vi "Plot Loop.vi"(8 "error in":errorcluster, 9 "Cluster Of Graphs":T2, 10 "Reference For PLot":T3) -> (0 "error out":errorcluster)   [LabVIEW 2015]
uses:
  TypeDef/UE Reference For Plot.ctl
  TypeDef/Plot Cluster.ctl
  TypeDef/GraphReff.ctl
panel:
  in  "InitializationValue-Input-PieCahrt":T1={"InitializationDefect"=[0.0, 0.0, 0.0, 0.0, 0.0, 0.0, 0.0, 0.0, 0.0, 0.0, 0.0, 0.0, 0.0, 0.0, 0.0, 0.0, 0.0, 0.0, 0.0, 0.0, 0.0, 0.0, 0.0, 0.0, 0.0, 0.0, 0.0, 0.0, 0.0, 0.0, 0.0, 0.0, 0.0, 0.0, 0.0, 0.0, 0.0, 0.0, 0.0, 0.0], "InitializationProduction"=[0.0, 0.0, 0.0, 0.0, 0.0, 0.0, 0.0]}
  in  "InitializationValue-Input-Barplot":T1={"InitializationDefect"=[0.0, 0.0, 0.0, 0.0, 0.0, 0.0, 0.0, 0.0, 0.0, 0.0, 0.0, 0.0, 0.0, 0.0, 0.0, 0.0, 0.0, 0.0, 0.0, 0.0, 0.0, 0.0, 0.0, 0.0, 0.0, 0.0, 0.0, 0.0, 0.0, 0.0, 0.0, 0.0, 0.0, 0.0, 0.0, 0.0, 0.0, 0.0, 0.0, 0.0, 0.0], "InitializationProduction"=[0.0, 0.0, 0.0, 0.0, 0.0, 0.0]}
  # "Plot Loop Test Bench"
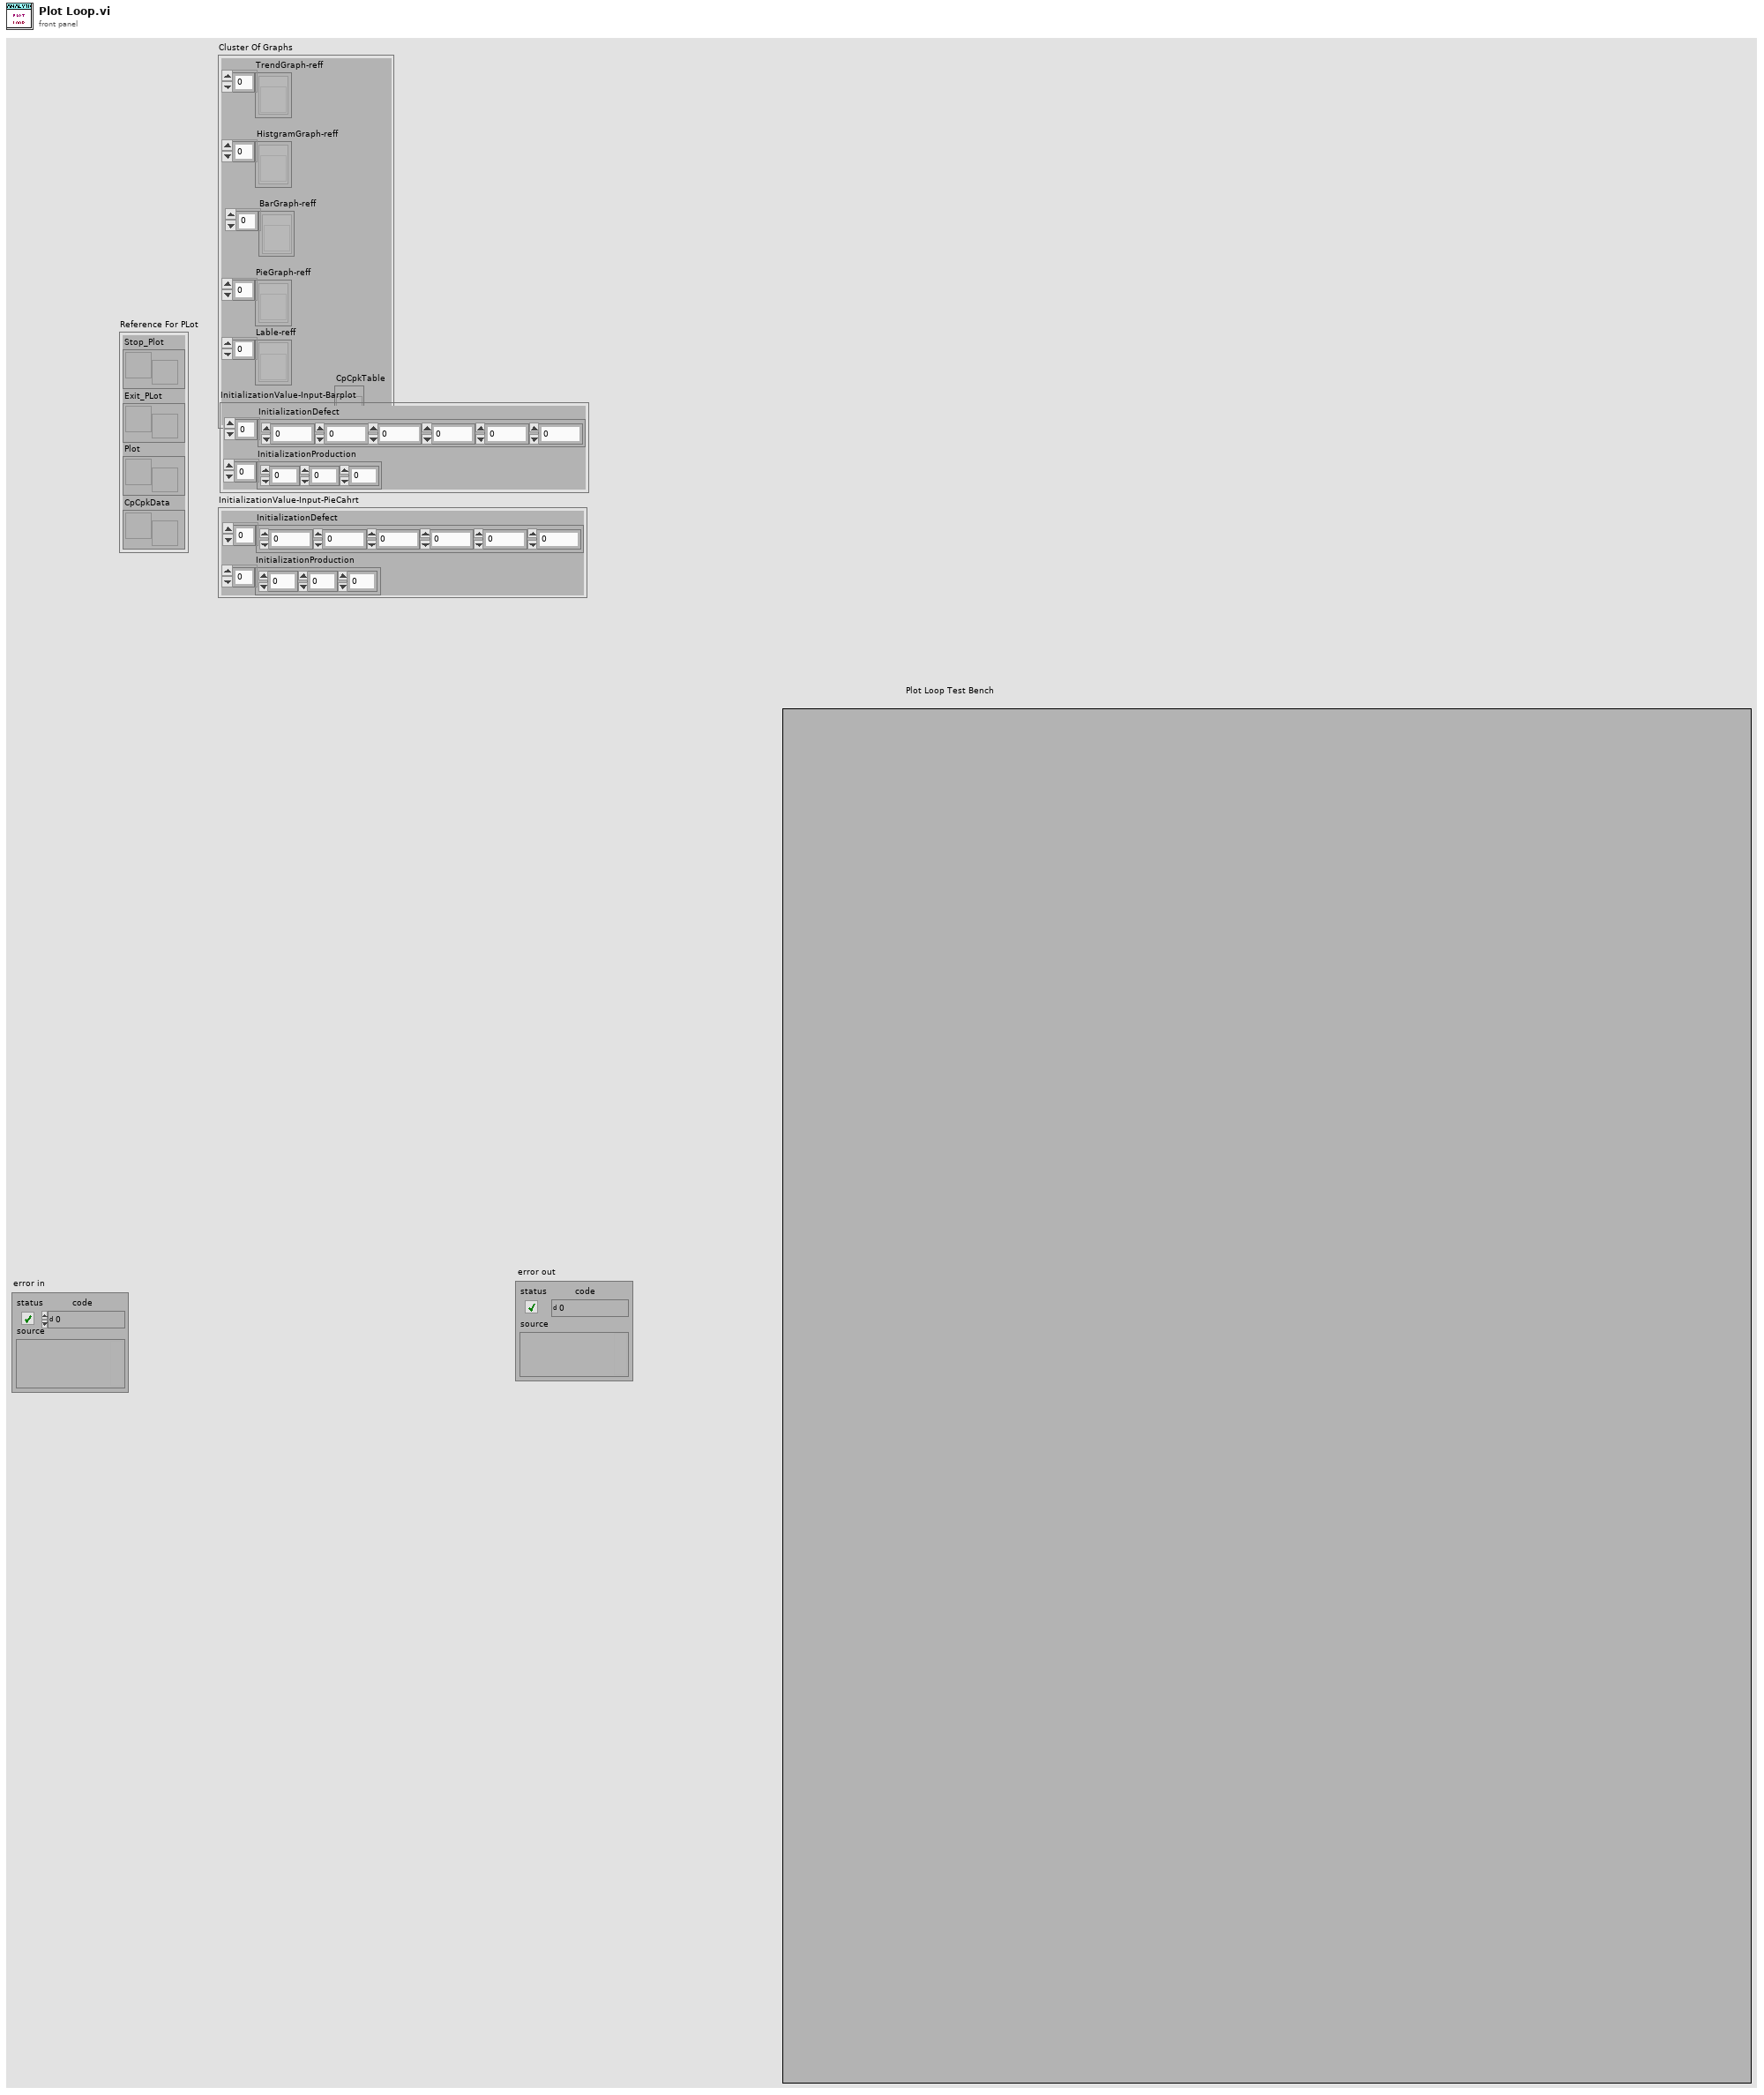
[diagram p1: front panel]
types:
  T1 = cluster{"InitializationDefect":dbl[], "InitializationProduction":dbl[]}
  T2 = typedef "GraphReff.ctl" = cluster{"HistgramGraph-reff":refnum<vi>[], "BarGraph-reff":refnum<vi>[], "PieGraph-reff":refnum<vi>[], "Lable-reff":refnum<vi>[], "TrendGraph-reff":refnum<vi>[], "CpCpkTable":refnum<vi>}
  T3 = typedef "UE Reference For Plot.ctl" = cluster{"Stop_Plot":refnum<user-event>, "Exit_PLot":refnum<user-event>, "Plot":refnum<user-event>, "CpCpkData":refnum<user-event>}
  T4 = enum32{"invalid app kind", "Development System", "Run Time System", "Student Edition", "Embedded LabVIEW", "Evaluation", "Custom"}
  T5 = enum32{"Invalid", "Standard", "Closed", "Hidden", "Minimized", "Maximized"}
  T6 = typedef "Plot Cluster.ctl" = cluster{"Reduced 2D":dbl[][], "Start Index":i32, "MeasurementData":cluster{"MeasurementID":i32, "MeasureEnable":bool, "MeasurementPass":bool, "LimitSets":cluster{"LimitSetId":i32, "Limits":dbl[]}[]}[], "No Of New Termnals":i32, "Top/Bottom":bool, "Values Inserted":i32, "PlotParameters":cluster{"Trend":cluster{"TrendID":i32, "PlotEnable":bool, "PlotTitle":string, "PlotCaptionFont":cluster{"FontName":string, "FontSize":i32, "IsBold":bool, "IsItalic":bool, "IsUnderline":bool, "IsStrikeout":bool, "FontColor":string}, "XLabel":string, "XLabelFont":cluster{"FontName":string, "FontSize":i32, "IsBold":bool, "IsItalic":bool, "IsUnderline":bool, "IsStrikeout":bool, "FontColor":string}, "SamplesToDisplay":i32, "Channels":cluster{"Label":string, "YLabelFont":cluster{"FontName":string, "FontSize":i32, "IsBold":bool, "IsItalic":bool, "IsUnderline":bool, "IsStrikeout":bool, "FontColor":string}, "MeasurementID":i32, "PlotColor":string, "PointShape":string, "ShowOnGraph":bool}[]}[], "Histogram":cluster{"HistogramID":i32, "PlotEnable":bool, "PlotTitle":string, "PlotLabelFont":cluster{"FontName":string, "FontSize":i32, "IsBold":bool, "IsItalic":bool, "IsUnderline":bool, "IsStrikeout":bool, "FontColor":string}, "XLabel":string, "XLabelFont":cluster{"FontName":string, "FontSize":i32, "IsBold":bool, "IsItalic":bool, "IsUnderline":bool, "IsStrikeout":bool, "FontColor":string}, "YLabel":string, "YLabelFont":cluster{"FontName":string, "FontSize":i32, "IsBold":bool, "IsItalic":bool, "IsUnderline":bool, "IsStrikeout":bool, "FontColor":string}, "MeasurementID":i32, "PlotColor":string, "SamplesToDisplay":i32}[], "BarPlot":cluster{"BarPlotID":i32, "BarValuesID":i32, "PlotEnable":bool, "PlotLabel":string, "PlotLabelFont":cluster{"FontName":string, "FontSize":i32, "IsBold":bool, "IsItalic":bool, "IsUnderline":bool, "IsStrikeout":bool, "FontColor":string}, "XLabel":string, "XLabelFont":cluster{"FontName":string, "FontSize":i32, "IsBold":bool, "IsItalic":bool, "IsUnderline":bool, "IsStrikeout":bool, "FontColor":string}, "YLabel":string, "YLabelFont":cluster{"FontName":string, "FontSize":i32, "IsBold":bool, "IsItalic":bool, "IsUnderline":bool, "IsStrikeout":bool, "FontColor":string}, "Sectors":string[]}[], "PieChart":cluster{"PieChartID":i32, "PieChartValueID":i32, "PlotEnable":bool, "PlotLabel":string, "PlotLabelFont":cluster{"FontName":string, "FontSize":i32, "IsBold":bool, "IsItalic":bool, "IsUnderline":bool, "IsStrikeout":bool, "FontColor":string}, "Sectors":string[]}[]}, "Re-Initialised":bool, "Statistical params":string[][], "MeasurementData_IndexValues":cluster{"Measurement-ID":i32[], "Measurement-Enable":bool[], "LSL":dbl[], "USL":dbl[]}}
  T7 = cluster{"MeasurementID":i32, "MeasureEnable":bool, "MeasurementPass":bool, "LimitSets":cluster{"LimitSetId":i32, "Limits":dbl[]}[]}[]
  T8 = cluster{"Trend":cluster{"TrendID":i32, "PlotEnable":bool, "PlotTitle":string, "PlotCaptionFont":cluster{"FontName":string, "FontSize":i32, "IsBold":bool, "IsItalic":bool, "IsUnderline":bool, "IsStrikeout":bool, "FontColor":string}, "XLabel":string, "XLabelFont":cluster{"FontName":string, "FontSize":i32, "IsBold":bool, "IsItalic":bool, "IsUnderline":bool, "IsStrikeout":bool, "FontColor":string}, "SamplesToDisplay":i32, "Channels":cluster{"Label":string, "YLabelFont":cluster{"FontName":string, "FontSize":i32, "IsBold":bool, "IsItalic":bool, "IsUnderline":bool, "IsStrikeout":bool, "FontColor":string}, "MeasurementID":i32, "PlotColor":string, "PointShape":string, "ShowOnGraph":bool}[]}[], "Histogram":cluster{"HistogramID":i32, "PlotEnable":bool, "PlotTitle":string, "PlotLabelFont":cluster{"FontName":string, "FontSize":i32, "IsBold":bool, "IsItalic":bool, "IsUnderline":bool, "IsStrikeout":bool, "FontColor":string}, "XLabel":string, "XLabelFont":cluster{"FontName":string, "FontSize":i32, "IsBold":bool, "IsItalic":bool, "IsUnderline":bool, "IsStrikeout":bool, "FontColor":string}, "YLabel":string, "YLabelFont":cluster{"FontName":string, "FontSize":i32, "IsBold":bool, "IsItalic":bool, "IsUnderline":bool, "IsStrikeout":bool, "FontColor":string}, "MeasurementID":i32, "PlotColor":string, "SamplesToDisplay":i32}[], "BarPlot":cluster{"BarPlotID":i32, "BarValuesID":i32, "PlotEnable":bool, "PlotLabel":string, "PlotLabelFont":cluster{"FontName":string, "FontSize":i32, "IsBold":bool, "IsItalic":bool, "IsUnderline":bool, "IsStrikeout":bool, "FontColor":string}, "XLabel":string, "XLabelFont":cluster{"FontName":string, "FontSize":i32, "IsBold":bool, "IsItalic":bool, "IsUnderline":bool, "IsStrikeout":bool, "FontColor":string}, "YLabel":string, "YLabelFont":cluster{"FontName":string, "FontSize":i32, "IsBold":bool, "IsItalic":bool, "IsUnderline":bool, "IsStrikeout":bool, "FontColor":string}, "Sectors":string[]}[], "PieChart":cluster{"PieChartID":i32, "PieChartValueID":i32, "PlotEnable":bool, "PlotLabel":string, "PlotLabelFont":cluster{"FontName":string, "FontSize":i32, "IsBold":bool, "IsItalic":bool, "IsUnderline":bool, "IsStrikeout":bool, "FontColor":string}, "Sectors":string[]}[]}
  T9 = cluster{"Measurement-ID":i32[], "Measurement-Enable":bool[], "LSL":dbl[], "USL":dbl[]}
  T10 = cluster{"Core":cluster{"Current VI Reference":refnum<vi>, "Close Panel on Exit?":bool}, "Plot-data":T6}
  T11 = cluster{"Current VI Reference":refnum<vi>, "Close Panel on Exit?":bool}
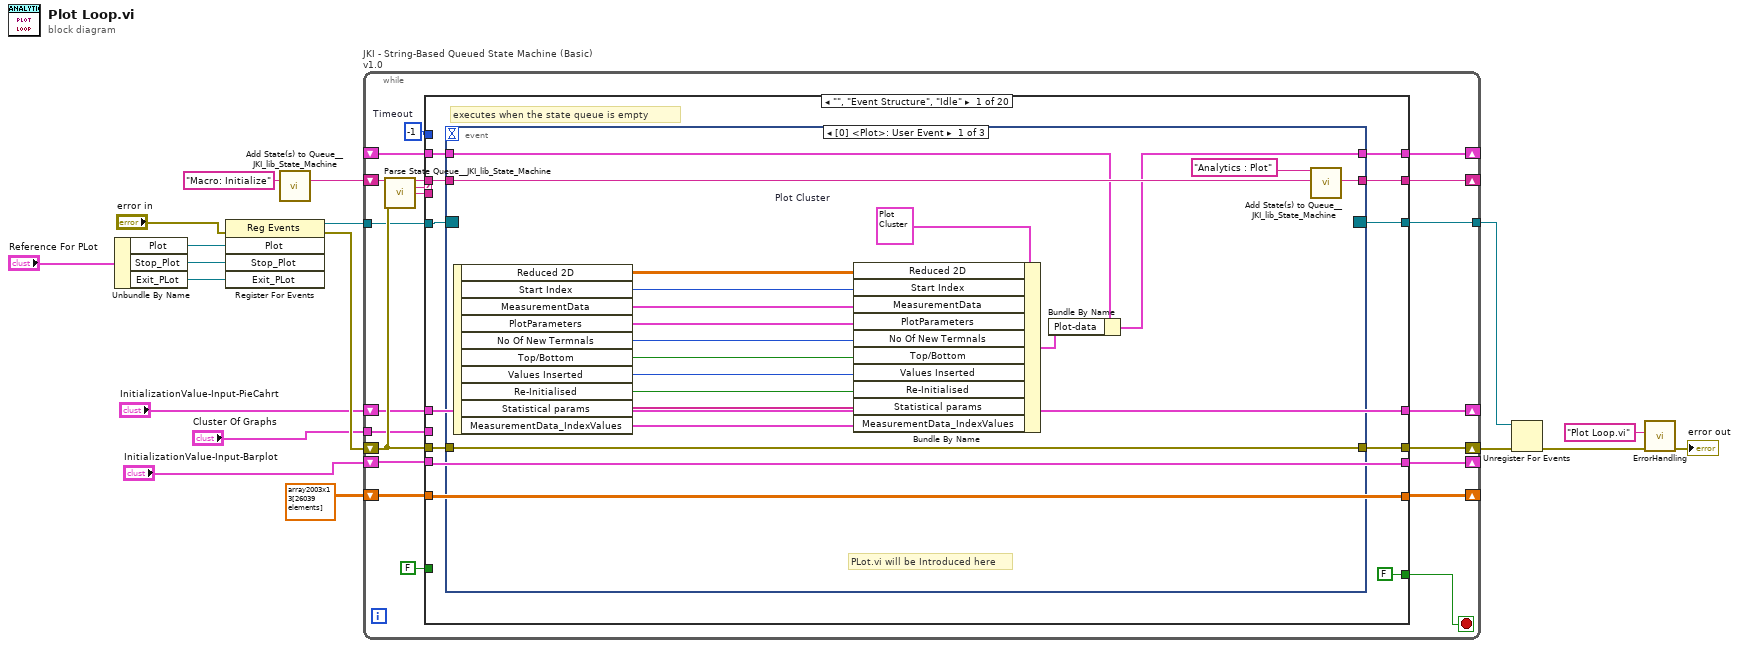
[diagram p0: block diagram]
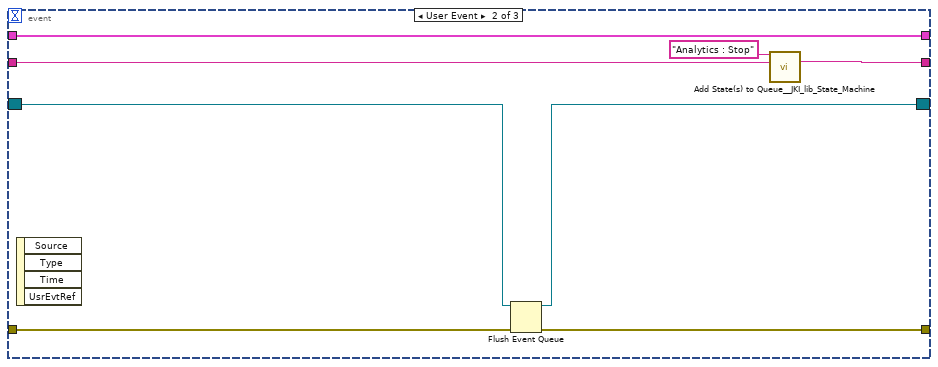
[diagram p2: hidden frame]
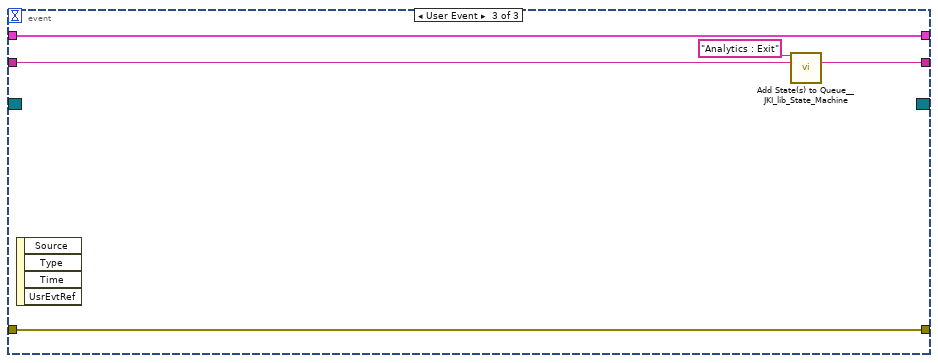
[diagram p3: hidden frame]
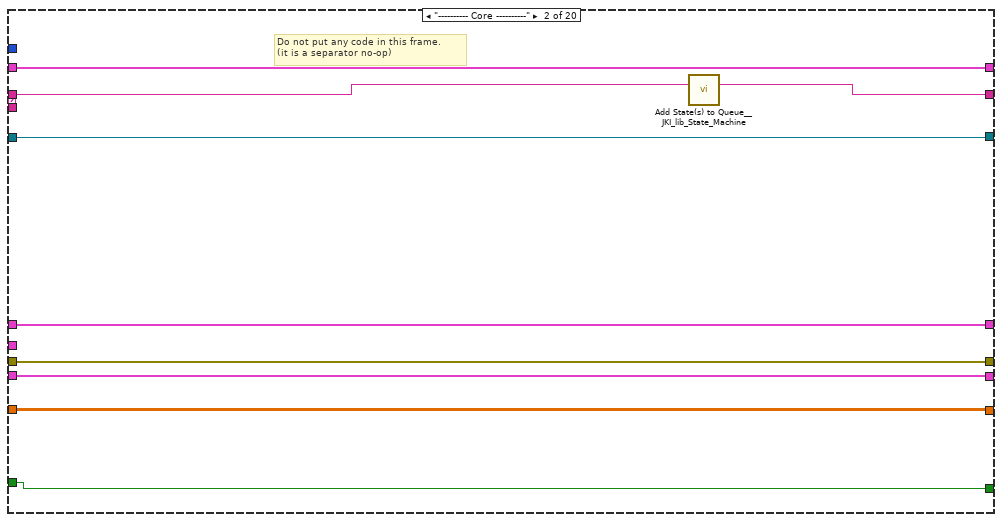
[diagram p4: hidden frame]
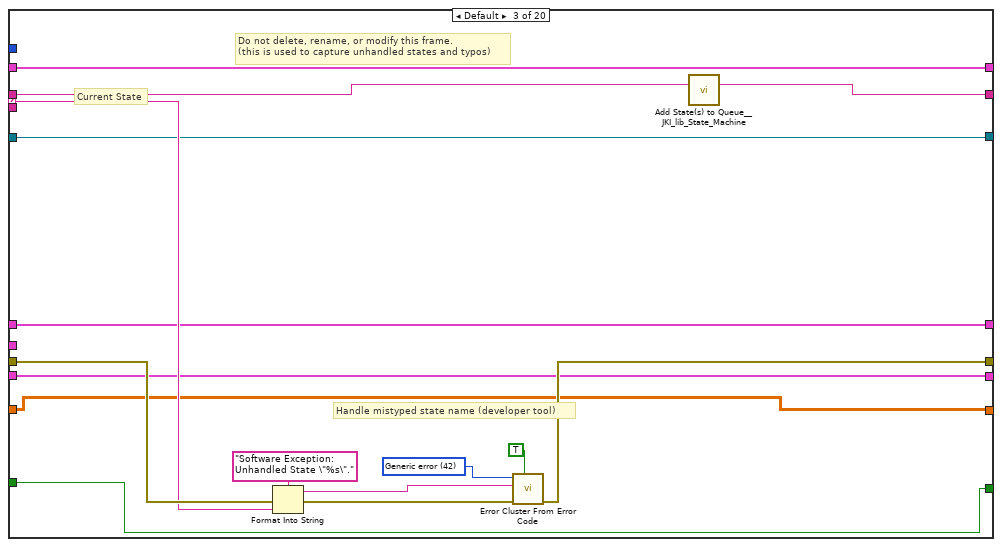
[diagram p5: hidden frame]
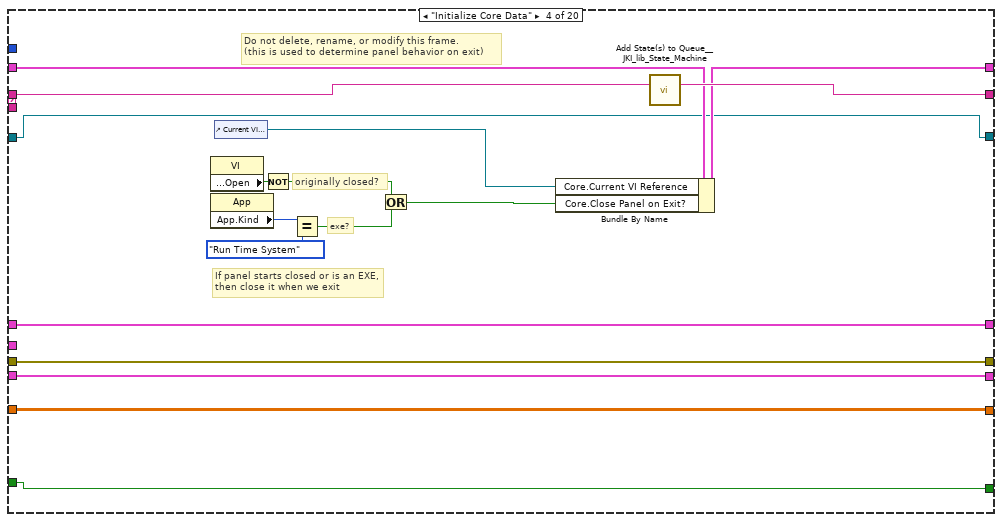
[diagram p6: hidden frame]
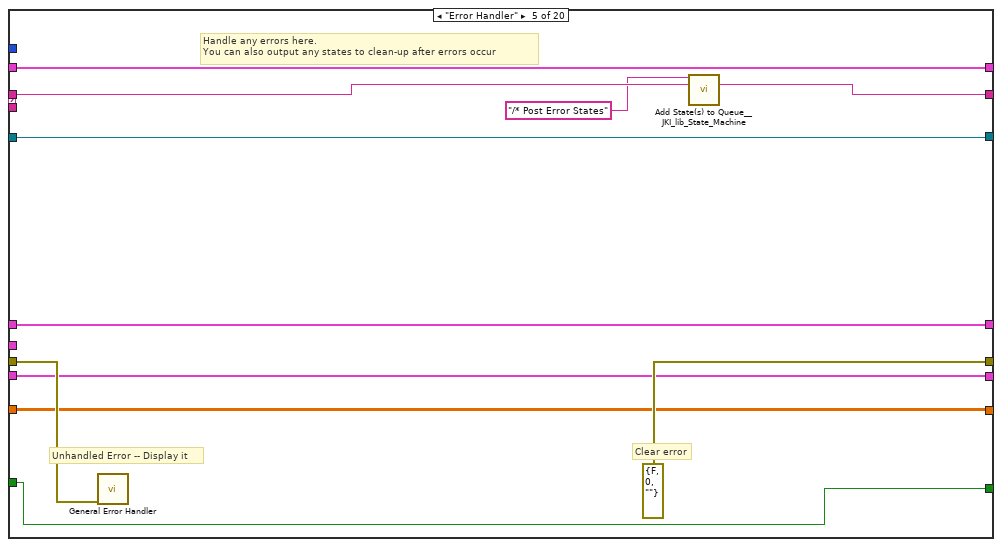
[diagram p7: hidden frame]
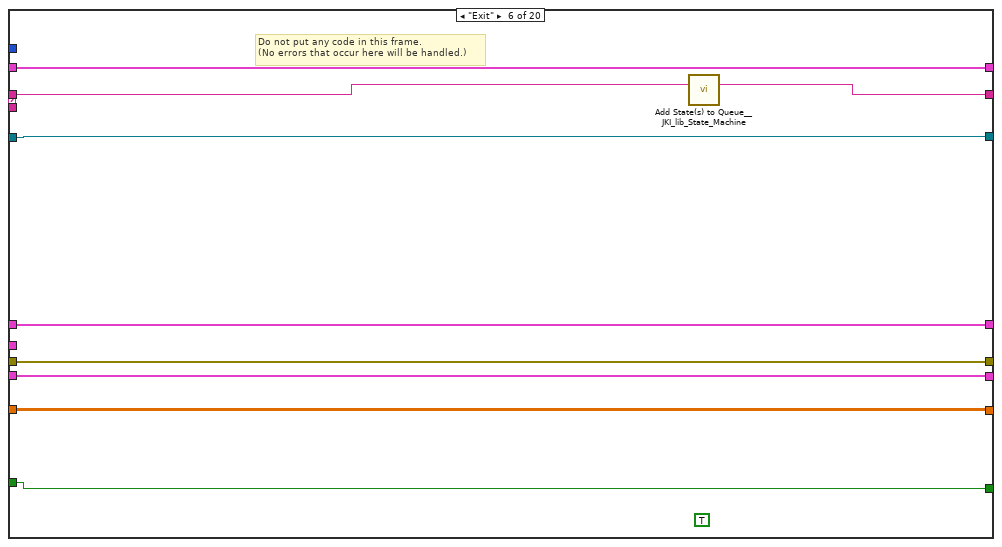
[diagram p8: hidden frame]
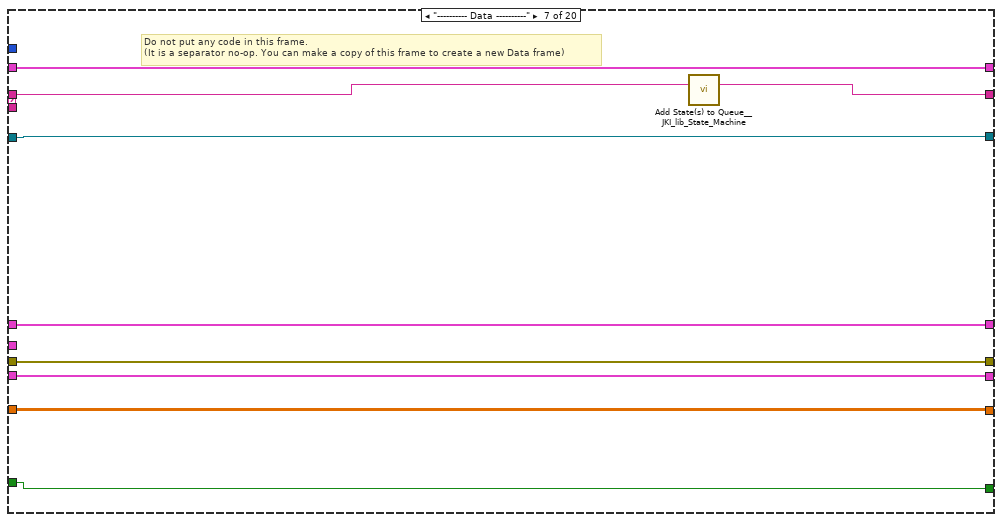
[diagram p9: hidden frame]
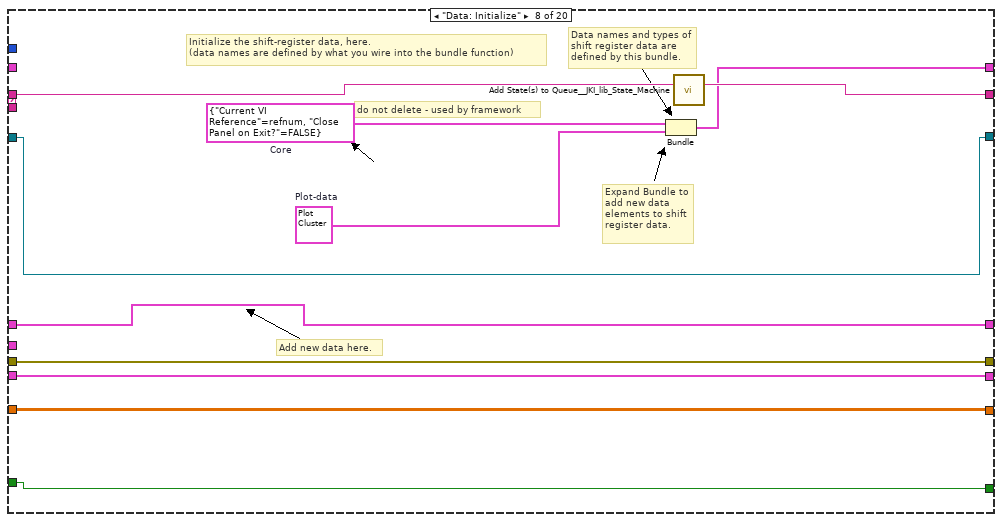
[diagram p10: hidden frame]
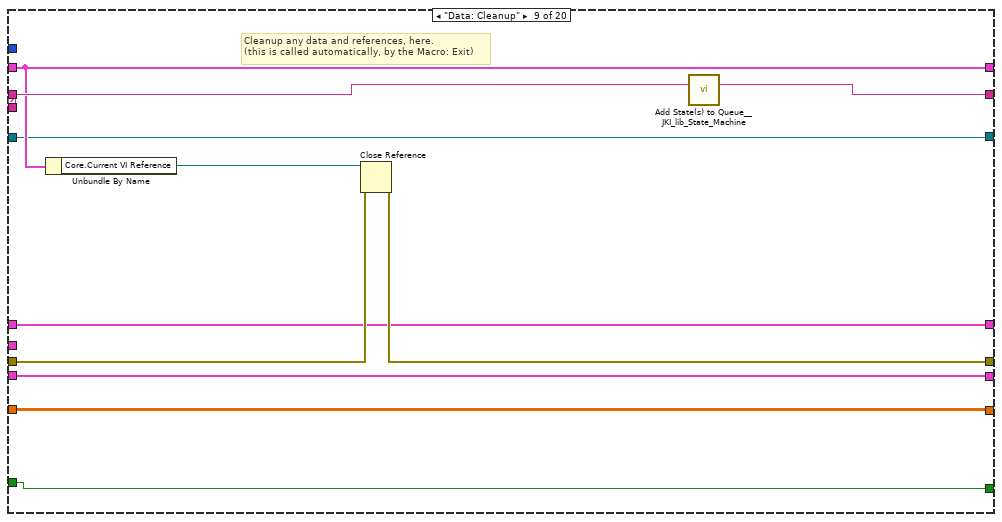
[diagram p11: hidden frame]
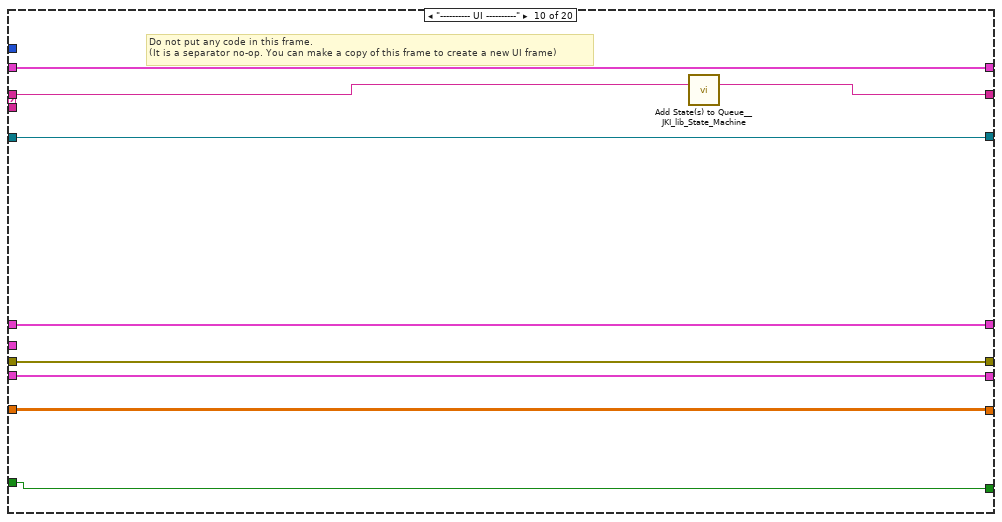
[diagram p12: hidden frame]
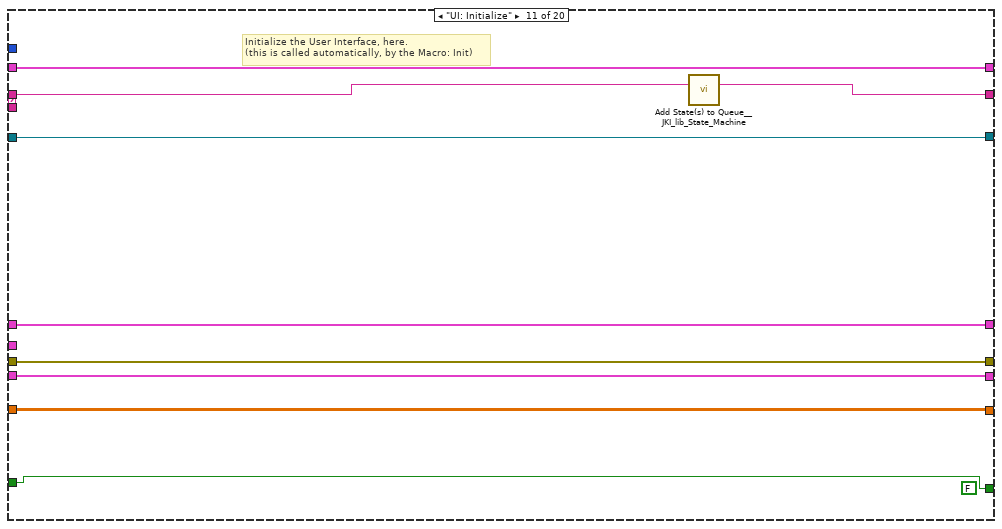
[diagram p13: hidden frame]
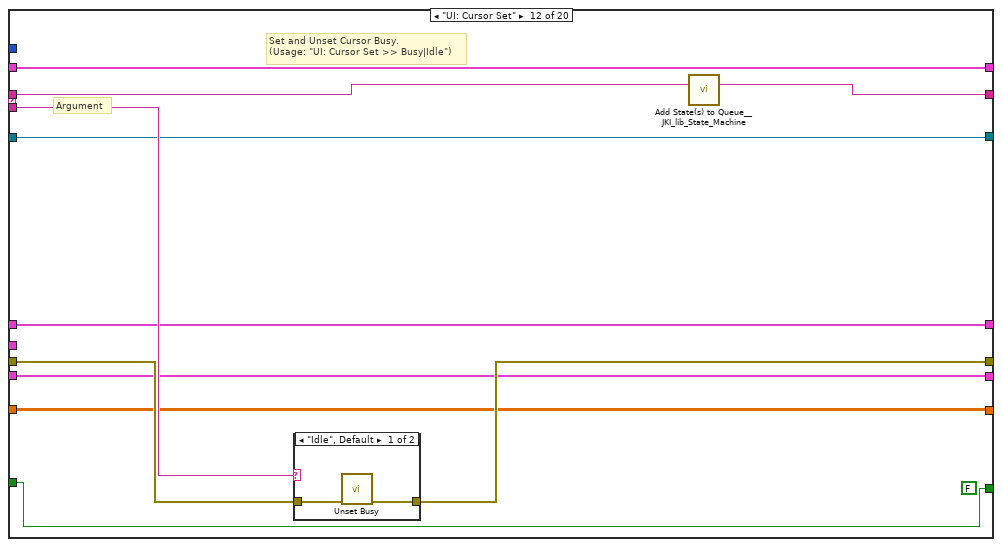
[diagram p14: hidden frame]
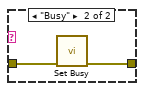
[diagram p15: hidden frame]
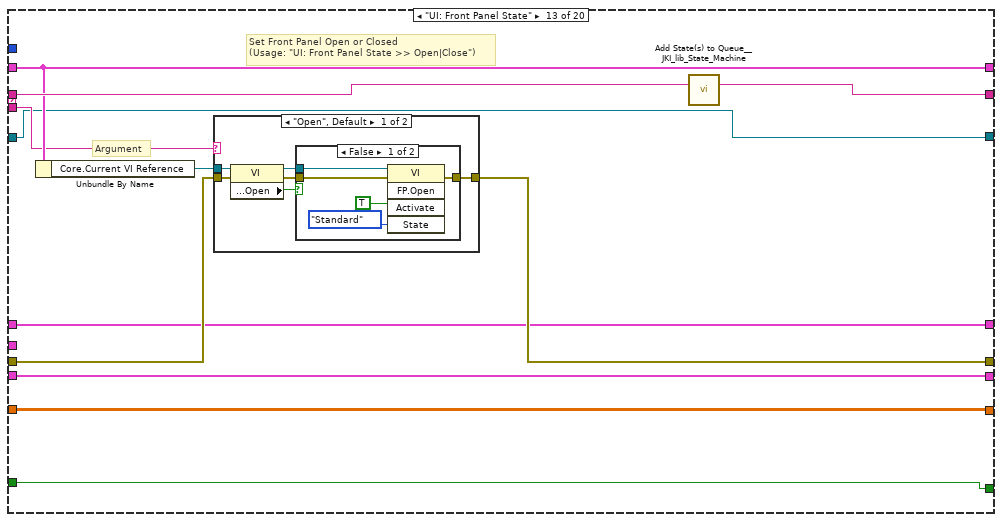
[diagram p16: hidden frame]
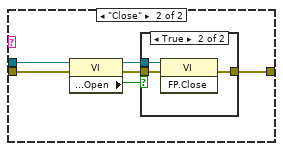
[diagram p18: hidden frame]
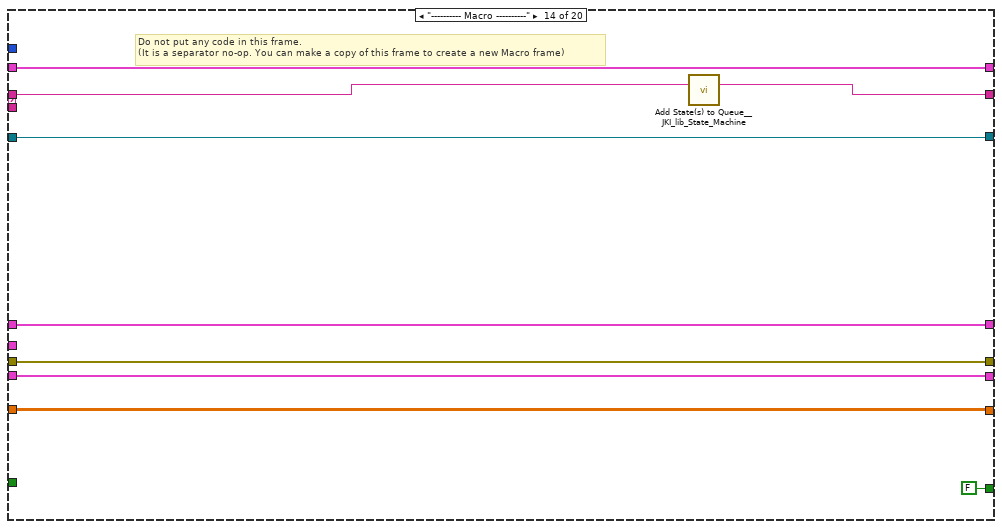
[diagram p20: hidden frame]
diagram:
  n1 = Unbundle By Name("Reference For PLot") -> ("Plot"=w11:refnum<user-event>, "Stop_Plot"=w15:refnum<user-event>, "Exit_PLot"=w14:refnum<user-event>)
  n2 = register-events(error in="error in", w11, w15, w14) -> (reference out=w8:refnum<event-registration>, error out=w7:errorcluster)  [unwired: 1 in]
  n3 = call <vilib>:"Add State(s) to Queue__JKI_lib_State_Machine.vi"("State(s) in (\"\")"="Macro: Initialize") -> ("States Out"=w10:string)  [unwired: 14 in]
  n4 = while "JKI - String-Based Queued State Machine (Basic) v1.0" {
    shift-right: [w33] -> _
    shift-left: _ -> [w32]
    shift-right: [w35] -> w2
    shift-left: w7 -> [w30]
    shift-right: [w34] -> _
    shift-left: w10 -> [w36]
    tunnel: w8 -> [w29]
    tunnel: "Cluster Of Graphs" -> [w26]
    tunnel: [w24] -> w1
    shift-right: [w22] -> _
    shift-left: "InitializationValue-Input-PieCahrt" -> [w25]
    shift-right: [w21] -> _
    shift-left: "InitializationValue-Input-Barplot" -> [w27]
    shift-right: [w23] -> _
    shift-left: dbl[][] array2003x13[26039 elements] ("Initialization input") -> [w28]
    stop <- w20 stop-if-true
    w31 = -1  # Timeout
    n5 = call <vilib>:"Parse State Queue__JKI_lib_State_Machine.vi"("State Queue"=w36, "Error In (no error)"=w30) -> ("Remaining States"=w38:string, "Current State"=w39:string, "Arguments"=w37:string)  [unwired: 11 in]
    n6 = case shown="\"\", \"Event Structure\", \"Idle\"" w39 {
      selector: w39 -> [_ _ w97 _ _ _ _ _ _ _ _ _ _ _ _ _ _ _ _ _]
      tunnel: w38 -> [w48 w91 w101 w124 w135 w144 w153 w164 w175 w184 w193 w204 w220 w251 w261 w276 w285 w300 w308 w310]
      tunnel: w37 -> [_ _ _ _ _ _ _ _ _ _ _ w199 w214 _ _ _ _ _ _ _]
      tunnel: w32 -> [w45 w88 w99 w115 w132 w142 w150 _ w170 w181 w191 w202 w216 w248 w258 w273 w282 w297 w305 w318]
      tunnel: [w50 w89 w103 w121 errorcluster {"status"=FALSE, "code"=0, "source"=""} ("error out") w141 w151 w161 w171 w182 w190 w200 w217 w249 w259 w274 w283 w295 w306 w315] -> w35
      tunnel: w30 -> [w51 w89 w102 w121 w131 w141 w151 w161 w172 w182 w190 w201 w218 w249 w259 w274 w283 w296 w306 w316]
      tunnel: [w47 w90 w100 w123 w134 w143 w152 w163 w174 w183 w192 w203 w219 w250 w260 w275 w284 w299 w307 w309] -> w34
      tunnel: [w46 w88 w99 w122 w132 w142 w150 w162 w170 w181 w191 w202 w216 w248 w258 w273 w282 w297 w305 w318] -> w33
      tunnel: w31 -> [_ _ _ _ _ _ _ _ _ _ _ _ _ _ _ _ _ _ _ _]
      tunnel: w29 -> [w49 w87 w96 w112 w129 w140 w149 w159 w169 w180 w189 w198 w213 w247 w256 w266 w281 w298 w304 w317]
      tunnel: w28 -> [w41 w84 w93 w109 w126 w137 w146 w155 w166 w177 w186 w195 w210 w244 w253 w263 w278 w291 _ _]
      tunnel: w27 -> [w40 w85 w94 w110 w127 w138 w147 w156 w167 w178 w187 w196 w211 w245 w254 w264 w279 w290 _ _]
      tunnel: w26 -> [_ _ _ _ _ _ _ _ _ _ _ _ _ _ _ _ _ w292 _ w314]
      tunnel: w25 -> [w42 w86 w95 w111 w128 w139 w148 w157 w168 w179 w188 w197 w212 w246 w255 w265 w280 w293 _ _]
      tunnel: [w44 w87 w96 w112 w129 w140 w149 w159 w169 w180 w189 w198 w213 w247 w256 w266 w281 w298 w304 w317] -> w24
      tunnel: [w41 w84 w93 w109 w126 w137 w146 w155 w166 w177 w186 w195 w210 w244 w253 w263 w278 w289 dbl[][] array2001x13[26013 elements] ("Initialization input") dbl[][] array2001x13[26013 elements] ("Initialization input")] -> w23
      tunnel: [w42 w86 w95 w111 w128 w139 w148 w157 w168 w179 w188 w197 w212 w246 w255 w265 w280 w288 w302 w313] -> w22
      tunnel: [w40 w85 w94 w110 w127 w138 w147 w156 w167 w178 w187 w196 w211 w245 w254 w264 w279 w287 w302 w313] -> w21
      tunnel: [FALSE w83 w92 w108 w125 w136 w145 w154 w165 w176 w185 w194 w209 FALSE FALSE TRUE FALSE FALSE FALSE TRUE] -> w20
      tunnel: FALSE -> [_ w83 w92 w108 w125 w136 w145 w154 w165 w176 w185 w194 w209 _ _ _ _ _ _ _]
      frame "", "Event Structure", "Idle" {
        # "executes when the state queue is empty"
        n7 = event shown="[0] <Plot>: User Event" {
          selector: w49 -> [_ w75 _]
          dyn-events: [_ w74 _] -> w44
          timeout: _ -> [_ _ _]
          tunnel: w51 -> [w57 w77 w78]
          tunnel: [w57 w76 w78] -> w50
          tunnel: w48 -> [w60 w71 w80]
          tunnel: [w59 w72 w81] -> w47
          tunnel: [w54 w73 w82] -> w46
          tunnel: w45 -> [w56 w73 w82]
          event User Event {
            w65 = T6 {"Reduced 2D"=[], "Start Index"=0, "MeasurementData"=[], "No Of New Termnals"=0, "Top/Bottom"=FALSE, "Values Inserted"=0, "PlotParameters"={"Trend"=[], "Histogram"=[], "BarPlot"=[], "PieChart"=[]}, "Re-Initialised"=FALSE, "Statistical params"=[], "MeasurementData_IndexValues"={"Measurement-ID"=[], "Measurement-Enable"=[], "LSL"=[], "USL"=[]}}  # Plot Cluster
            # "PLot.vi will be Introduced here"
            n8 = event-data() -> ("Reduced 2D"=w67:dbl[][], "Start Index"=w68:i32, "MeasurementData"=w66:T7, "PlotParameters"=w69:T8, "No Of New Termnals"=w64:i32, "Top/Bottom"=w63:bool, "Values Inserted"=w62:i32, "Re-Initialised"=w61:bool, "Statistical params"=w53:string[][], "MeasurementData_IndexValues"=w52:T9)  [unwired: 1 in]
            n9 = Bundle By Name(cluster=w65, "Reduced 2D"=w67, "Start Index"=w68, "MeasurementData"=w66, "PlotParameters"=w69, "No Of New Termnals"=w64, "Top/Bottom"=w63, "Values Inserted"=w62, "Re-Initialised"=w61, "Statistical params"=w53, "MeasurementData_IndexValues"=w52) -> (w55:T6)
            n10 = Bundle By Name(cluster=w56, "Plot-data"=w55) -> (w54:T10)
            n11 = call <vilib>:"Add State(s) to Queue__JKI_lib_State_Machine.vi"("State(s) in Front (\"\")"="Analytics : Plot" ("State(s) in Front (\"\")"), "State(s) in (\"\")"=w60) -> ("States Out"=w59:string)  [unwired: 13 in]
          }
          event User Event {
            n12 = event-data() -> ()  [unwired: 1 in, 4 out]
            n13 = Flush Event Queue(0:w75, 3:w77) -> (8:w74:refnum<event-registration>, 11:w76:errorcluster)  [unwired: 4 in, 1 out]
            n14 = call <vilib>:"Add State(s) to Queue__JKI_lib_State_Machine.vi"("State(s) in Front (\"\")"="Analytics : Stop" ("State(s) in Front (\"\")"), "State(s) in (\"\")"=w71) -> ("States Out"=w72:string)  [unwired: 13 in]
          }
          event User Event {
            n15 = event-data() -> ()  [unwired: 1 in, 4 out]
            n16 = call <vilib>:"Add State(s) to Queue__JKI_lib_State_Machine.vi"("State(s) in Front (\"\")"="Analytics : Exit" ("State(s) in Front (\"\")"), "State(s) in (\"\")"=w80) -> ("States Out"=w81:string)  [unwired: 13 in]
          }
        }
      }
      frame "---------- Core ----------" {
        # "Do not put any code in this frame.\n(it is a separator no-op)"
        n17 = call <vilib>:"Add State(s) to Queue__JKI_lib_State_Machine.vi"("State(s) in (\"\")"=w91) -> ("States Out"=w90:string)  [unwired: 14 in]
      }
      frame Default {
        w106 = 42 items=["No error", "Argument error", "Memory is full", "Out of zone", "End of file", "File already open", "Generic file I/O error", "File not found", "File permission error", "Disk is full", "Duplicate path", "Too many files open", "System feature not enabled", "Resource file not found", "Cannot add resource", "Resource not found", "Image not found", "Image memory error", "Pen does not exist", "Config type invalid", "Config token not found", "Config parse error", "Config memory error", "Bad external code format", "Bad external code offset", "External code not present", "Null window", "Destroy window error", "Null menu", "Print aborted", "Bad print record", "Print driver error", "Windows error during printing", "Memory error during printing", "Print dialog error", "Generic print error", "Invalid device refnum", "Device not found", "Device parameter error", "Device unit error", "Cannot open device", "Device call aborted", "Generic error", "Cancelled by user", "Object ID too low", "Object ID too high", "Object not in heap", "Unknown heap", "Unknown object (invalid DefProc)", "Unknown object (DefProc not in table)", "Message out of range", "Invalid (null) method", "Unknown message", "Manager call not supported", "Bad address", "Network operation in progress", "Network operation timed out", "Connection is busy", "Network attribute not supported", "Network error", "Address in use", "System out of memory", "Connection aborted", "Connection refused", "Not connected", "Already connected", "Connection closed", "Initialization error (interapplication manager)", "Bad occurrence", "Wait on unbound occurrence handler", "Occurrence queue overflow", "Datalog type conflict", "Unused", "Unrecognized type (interapplication manager)", "Memory corrupt", "Failed to make temporary DLL", "Old CIN version", "Drag socket not found", "Failed to load drop-object", "Failed to register OLE object", "Failed to release OLE object", "Format specifier type mismatch", "Unknown format specifier", "Too few format specifiers", "Too many format specifiers", "Scan failed", "Newer CIN version", "Error converting to variant", "Runtime menu error", "Password tampered", "Variant attribute not found", "Incompatible variant data type", "Event data is not available", "Event Store is not present", "Occurrence is not found", "Event Queue is not created", "Event info is not available", "Refnum passed is NULL", "Error retrieving Class GUID", "Error retrieving CoClass GUID", "Error retrieving TypeLib GUID.", "Bad built application magic bytes.", "Specific driver is different from the specific driver associated with the Logical Name.", "There is no session opened to the class driver.", "Max Error", "MAX - Error with config objects", "MAX - Error loading configuration", "MAX - Group not supported"]
        # "Current State"
        # "Do not delete, rename, or modify this frame.\n(this is used to capture unhandled states and typos)"
        # "Handle mistyped state name (developer tool)"
        n18 = Format Into String(format string="Software Exception: Unhandled State \"%s\"." ("message"), error in=w102, w97) -> (resulting string=w105:string, error out=w104:errorcluster)  [unwired: 1 in]
        n19 = call <vilib>:"Error Cluster From Error Code.vi"("show call chain? (False)"=TRUE, "error in (no error)"=w104, "error message (\"\")"=w105, "error code (0)"=w106) -> ("error out"=w103:errorcluster)  [unwired: 5 in]
        n20 = call <vilib>:"Add State(s) to Queue__JKI_lib_State_Machine.vi"("State(s) in (\"\")"=w101) -> ("States Out"=w100:string)  [unwired: 14 in]
      }
      frame "Initialize Core Data" {
        # "Do not delete, rename, or modify this frame.\n(this is used to determine panel behavior on exit)"
        # "originally closed?"
        # "exe?"
        # "If panel starts closed or is an EXE, then close it when we exit"
        n21 = property class="VI"() -> ("Front Panel.Open"=w120:bool)  [unwired: 2 in, 2 out]
        n22 = property class="App"() -> ("App.Kind"=w119:T4)  [unwired: 2 in, 2 out]
        n23 = control-ref of="Current VI Reference"() -> (w113:refnum<vi>)
        n24 = Not(x=w120) -> (.not. x?=w117:bool)
        n25 = Equal?(x=w119, y=T4."Run Time System" ("Application:Kind")) -> (x = y?=w116:bool)
        n26 = Or(x=w117, y=w116) -> (x .or. y?=w114:bool)
        n27 = Bundle By Name(cluster=w115, "Core.Current VI Reference"=w113, "Core.Close Panel on Exit?"=w114) -> (w122:T10)
        n28 = call <vilib>:"Add State(s) to Queue__JKI_lib_State_Machine.vi"("State(s) in (\"\")"=w124) -> ("States Out"=w123:string)  [unwired: 14 in]
      }
      frame "Error Handler" {
        # "Unhandled Error -- Display it"
        # "Handle any errors here.\nYou can also output any states to clean-up after errors occur"
        # "Clear error"
        n29 = call <vilib>:"General Error Handler.vi"("error in (no error)"=w131) -> ()  [unwired: 10 in, 5 out]
        n30 = call <vilib>:"Add State(s) to Queue__JKI_lib_State_Machine.vi"("State(s) in Front (\"\")"="/* Post Error States", "State(s) in (\"\")"=w135) -> ("States Out"=w134:string)  [unwired: 13 in]
      }
      frame "Exit" {
        (unwired) TRUE
        # "Do not put any code in this frame.\n(No errors that occur here will be handled.)"
        n31 = call <vilib>:"Add State(s) to Queue__JKI_lib_State_Machine.vi"("State(s) in (\"\")"=w144) -> ("States Out"=w143:string)  [unwired: 14 in]
      }
      frame "---------- Data ----------" {
        # "Do not put any code in this frame.\n(It is a separator no-op. You can make a copy of this frame to create a new Data frame)"
        n32 = call <vilib>:"Add State(s) to Queue__JKI_lib_State_Machine.vi"("State(s) in (\"\")"=w153) -> ("States Out"=w152:string)  [unwired: 14 in]
      }
      frame "Data: Initialize" {
        w158 = T6 {"Reduced 2D"=[], "Start Index"=0, "MeasurementData"=[], "No Of New Termnals"=0, "Top/Bottom"=FALSE, "Values Inserted"=0, "PlotParameters"={"Trend"=[], "Histogram"=[], "BarPlot"=[], "PieChart"=[]}, "Re-Initialised"=FALSE, "Statistical params"=[], "MeasurementData_IndexValues"={"Measurement-ID"=[], "Measurement-Enable"=[], "LSL"=[], "USL"=[]}}  # Plot-data
        w160 = T11 {"Current VI Reference"=refnum, "Close Panel on Exit?"=FALSE}  # Core
        # "do not delete - used by framework"
        # "Expand Bundle to add new data elements to shift register data."
        # "Add new data here."
        # "Data names and types of shift register data are defined by this bundle."
        # "Initialize the shift-register data, here.\n(data names are defined by what you wire into the bundle function)"
        n33 = Bundle("Core"=w160, "Plot-data"=w158) -> (w162:T10)  [unwired: 1 in]
        n34 = call <vilib>:"Add State(s) to Queue__JKI_lib_State_Machine.vi"("State(s) in (\"\")"=w164) -> ("States Out"=w163:string)  [unwired: 14 in]
      }
      frame "Data: Cleanup" {
        # "Cleanup any data and references, here.\n(this is called automatically, by the Macro: Exit)"
        n35 = Unbundle By Name(w170) -> ("Core.Current VI Reference"=w173:refnum<vi>)
        n36 = Close Reference(reference=w173, error in (no error)=w172) -> (error out=w171:errorcluster)
        n37 = call <vilib>:"Add State(s) to Queue__JKI_lib_State_Machine.vi"("State(s) in (\"\")"=w175) -> ("States Out"=w174:string)  [unwired: 14 in]
      }
      frame "---------- UI ----------" {
        # "Do not put any code in this frame.\n(It is a separator no-op. You can make a copy of this frame to create a new UI frame)"
        n38 = call <vilib>:"Add State(s) to Queue__JKI_lib_State_Machine.vi"("State(s) in (\"\")"=w184) -> ("States Out"=w183:string)  [unwired: 14 in]
      }
      frame "UI: Initialize" {
        (unwired) FALSE
        # "Initialize the User Interface, here.\n(this is called automatically, by the Macro: Init)"
        n39 = call <vilib>:"Add State(s) to Queue__JKI_lib_State_Machine.vi"("State(s) in (\"\")"=w193) -> ("States Out"=w192:string)  [unwired: 14 in]
      }
      frame "UI: Cursor Set" {
        (unwired) FALSE
        # "Argument"
        # "Set and Unset Cursor Busy.\n(Usage: \"UI: Cursor Set >> Busy|Idle\")"
        n40 = case shown="\"Idle\", Default" w199 {
          tunnel: w201 -> [w206 w208]
          tunnel: [w205 w207] -> w200
          frame "Idle", Default {
            n41 = call <vilib>:"Unset Busy.vi"("error in (no error)"=w206) -> ("error out"=w205:errorcluster)  [unwired: 10 in]
          }
          frame "Busy" {
            n42 = call <vilib>:"Set Busy.vi"("error in (no error)"=w208) -> ("error out"=w207:errorcluster)  [unwired: 9 in, 1 out]
          }
        }
        n43 = call <vilib>:"Add State(s) to Queue__JKI_lib_State_Machine.vi"("State(s) in (\"\")"=w204) -> ("States Out"=w203:string)  [unwired: 14 in]
      }
      frame "UI: Front Panel State" {
        # "Argument"
        # "Set Front Panel Open or Closed\n(Usage: \"UI: Front Panel State >> Open|Close\")"
        n44 = Unbundle By Name(w216) -> ("Core.Current VI Reference"=w215:refnum<vi>)
        n45 = case shown="\"Open\", Default" w214 {
          tunnel: w218 -> [w224 w237]
          tunnel: [w226 w238] -> w217
          tunnel: w215 -> [w225 w235]
          frame "Open", Default {
            n46 = property class="VI"(reference=w225, error in=w224) -> (reference out=w222:refnum<vi>, error out=w223:errorcluster, "Front Panel.Open"=w221:bool)
            n47 = case shown="False" w221 {
              tunnel: [w229 w232] -> w226
              tunnel: w223 -> [w228 w232]
              tunnel: w222 -> [w227 _]
              frame False {
                n48 = invoke class="VI" method="FP.Open"(reference=w227, error in=w228, "Activate"=TRUE, "State"=T5."Standard") -> (error out=w229:errorcluster)  [unwired: 1 in, 4 out]
              }
              frame True {
              }
            }
          }
          frame "Close" {
            n49 = property class="VI"(reference=w235, error in=w237) -> (reference out=w234:refnum<vi>, error out=w236:errorcluster, "Front Panel.Open"=w233:bool)
            n50 = case shown="True" w233 {
              tunnel: [w239 w242] -> w238
              tunnel: w236 -> [w239 w241]
              tunnel: w234 -> [_ w240]
              frame False {
              }
              frame True {
                n51 = invoke class="VI" method="FP.Close"(reference=w240, error in=w241) -> (error out=w242:errorcluster)  [unwired: 1 in, 2 out]
              }
            }
          }
        }
        n52 = call <vilib>:"Add State(s) to Queue__JKI_lib_State_Machine.vi"("State(s) in (\"\")"=w220) -> ("States Out"=w219:string)  [unwired: 14 in]
      }
      frame "---------- Macro ----------" {
        # "Do not put any code in this frame.\n(It is a separator no-op. You can make a copy of this frame to create a new Macro frame)"
        n53 = call <vilib>:"Add State(s) to Queue__JKI_lib_State_Machine.vi"("State(s) in (\"\")"=w251) -> ("States Out"=w250:string)  [unwired: 14 in]
      }
      frame "Macro: Initialize" {
        w257 = "Data: Initialize\nInitialize Core Data\nUI: Initialize\nUI: Front Panel State >> Close"  # Data: Initialize Initialize Core Data UI: Initialize UI: Front Panel State >> Close
        # "Initialization Macro\n(This is called once, when the VI starts)"
        n54 = call <vilib>:"Add State(s) to Queue__JKI_lib_State_Machine.vi"("State(s) in Front (\"\")"=w257, "State(s) in (\"\")"=w261) -> ("States Out"=w260:string)  [unwired: 13 in]
      }
      frame "Macro: Exit" {
        # "Exit Macro\n(This is called once, when the VI exits)"
        n55 = Unbundle By Name(w273) -> ("Core.Close Panel on Exit?"=w272:bool)
        n56 = Select(t="UI: Front Panel State >> Close", s=w272, f="") -> (s? t:f=w269:string)
        n57 = call <vilib>:"Add State(s) to Queue__JKI_lib_State_Machine.vi"("State(s) in (\"\")"=w269, "State(s) at Back (\"\")"="Data: Cleanup\nExit") -> ("States Out"=w267:string)  [unwired: 13 in]
        n58 = call <vilib>:"Add State(s) to Queue__JKI_lib_State_Machine.vi"("State(s) in Front (\"\")"=w267, "State(s) in (\"\")"=w276) -> ("States Out"=w275:string)  [unwired: 13 in]
      }
      frame "---------- Analytics----------" {
        # "Template Separator\n(You can make a copy of, or modify, this frame)"
        n59 = call <vilib>:"Add State(s) to Queue__JKI_lib_State_Machine.vi"("State(s) in (\"\")"=w285) -> ("States Out"=w284:string)  [unwired: 14 in]
      }
      frame "Analytics : Plot" {
        n60 = Unbundle By Name(w297) -> ("Plot-data"=w294:T6)
        n61 = call "Plot.vi"("InitializationValue-Input-Barplot"=w290, "InitializationValue-Input-PieCahrt"=w293, "error Input"=w296, "Initialization input"=w291, "Graph Refference's"=w292, "Plot Cluster"=w294) -> ("error output"=w295:errorcluster, "InitializationOutput"=w289:dbl[][], "InitializationValue-output-Barplot"=w287:T1, "InitializationValue-output-PieCahrt"=w288:T1)  [unwired: 2 in]
        n62 = call <vilib>:"Add State(s) to Queue__JKI_lib_State_Machine.vi"("State(s) in (\"\")"=w300) -> ("States Out"=w299:string)  [unwired: 14 in]
      }
      frame "Analytics : Stop" {
        w302 = T1 {"InitializationDefect"=[0.0, 0.0, 0.0, 0.0, 0.0, 0.0, 0.0, 0.0, 0.0, 0.0, 0.0, 0.0, 0.0, 0.0, 0.0, 0.0, 0.0, 0.0, 0.0, 0.0, 0.0, 0.0, 0.0, 0.0, 0.0, 0.0, 0.0, 0.0, 0.0, 0.0, 0.0, 0.0, 0.0, 0.0, 0.0, 0.0, 0.0, 0.0, 0.0, 0.0, 0.0], "InitializationProduction"=[0.0, 0.0, 0.0, 0.0, 0.0, 0.0, 0.0, 0.0, 0.0, 0.0, 0.0, 0.0, 0.0, 0.0, 0.0, 0.0, 0.0, 0.0, 0.0, 0.0, 0.0, 0.0, 0.0, 0.0, 0.0, 0.0, 0.0, 0.0, 0.0, 0.0, 0.0, 0.0, 0.0, 0.0, 0.0, 0.0, 0.0, 0.0, 0.0, 0.0, 0.0]} ("InitializationValue-output-PieCahrt")
        n63 = call <vilib>:"Add State(s) to Queue__JKI_lib_State_Machine.vi"("State(s) in (\"\")"=w308) -> ("States Out"=w307:string)  [unwired: 14 in]
      }
      frame "Analytics : Exit" {
        w313 = T1 {"InitializationDefect"=[0.0, 0.0, 0.0, 0.0, 0.0, 0.0, 0.0, 0.0, 0.0, 0.0, 0.0, 0.0, 0.0, 0.0, 0.0, 0.0, 0.0, 0.0, 0.0, 0.0, 0.0, 0.0, 0.0, 0.0, 0.0, 0.0, 0.0, 0.0, 0.0, 0.0, 0.0, 0.0, 0.0, 0.0, 0.0, 0.0, 0.0, 0.0, 0.0, 0.0, 0.0], "InitializationProduction"=[0.0, 0.0, 0.0, 0.0, 0.0, 0.0, 0.0, 0.0, 0.0, 0.0, 0.0, 0.0, 0.0, 0.0, 0.0, 0.0, 0.0, 0.0, 0.0, 0.0, 0.0, 0.0, 0.0, 0.0, 0.0, 0.0, 0.0, 0.0, 0.0, 0.0, 0.0, 0.0, 0.0, 0.0, 0.0, 0.0, 0.0, 0.0, 0.0, 0.0, 0.0]} ("InitializationValue-output-PieCahrt")
        n64 = call "Re-InitializaPlots.vi"("error in (no error)"=w316, "Cluster Of Graphs"=w314) -> ("error out"=w315:errorcluster)  [unwired: 9 in]
        n65 = call <vilib>:"Add State(s) to Queue__JKI_lib_State_Machine.vi"("State(s) in (\"\")"=w310) -> ("States Out"=w309:string)  [unwired: 14 in]
      }
    }
  }
  n66 = Unregister For Events(event registration refnum=w1, error in=w2) -> (error out=w17:errorcluster)
  n67 = call "ErrorHandling.vi"("error in (no error)"=w17, "Vi-name"="Plot Loop.vi") -> ("error out"=→"error out":errorcluster)  [unwired: 9 in]
